vi "store-can-data.vi"(4 "CAN frame":T2 {"payload" format="%x"; "timestamp" format="%<%.7X\n%x>T"; "type" items=["CAN Data"=0, "CAN Remote"=1, "CAN Bus Error"=2, "J1939 Data"=192, "Delay"=224, "Log Trigger"=225, "Start Trigger"=226]; "identifier" format="%x"}, 6 "id":u32 format="%.0x", 7 "child.tags":string[](array[string]), 8 "error in (no error)":errorcluster, 9 "tag":string, 10 "frame.type":T1, 11 "CANtable in":refnum<class "bAPPdata.lvclass">) -> (0 "error out":errorcluster, 3 "CANtable out":refnum<class "bAPPdata.lvclass">)   [LabVIEW 2015, in "bAPPdata.lvclass"]
uses:
  bAPPdata.lvclass
  <vilib>/xnet/xnet.llb/XNET Frame CAN.ctl
  <vilib>/xnet/xnet.llb/XNET Frame Type CAN.ctl
  subs/frame.type.ctl
  bAPPdata.lvclass/bAPPdata.ctl
  table-contents.ctl
  nMsgData.ctl
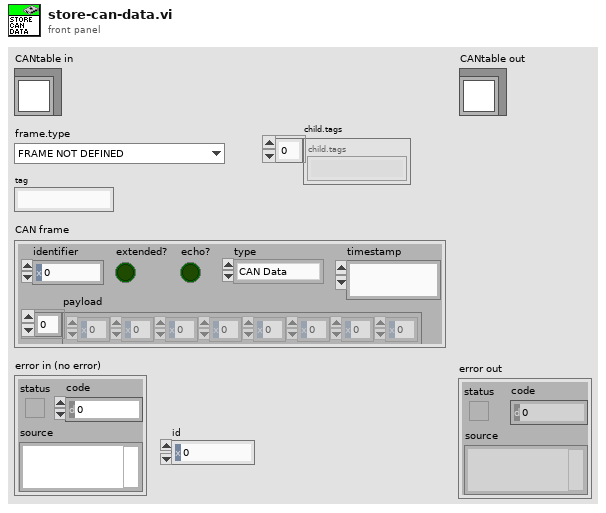
[diagram p1: front panel]
types:
  T1 = typedef "frame.type.ctl" = enum16{"FRAME NOT DEFINED", "DUT OUTPUT FRAME", "DUT INPUT FRAME"}
  T2 = typedef "XNET Frame CAN.ctl" = cluster{"timestamp":timestamp, "payload":u8[], "identifier":u32, "type":T3, "extended?":bool, "echo?":bool}
  T3 = typedef "XNET Frame Type CAN.ctl" = u8
  T4 = typedef "bAPPdata.lvclass/table-contents.ctl" = cluster{"id":u32, "tag":string, "frame.type":T1, "last.frame":T2, "tMsgData":T5, "child.tags":string[], "bit-payload":bool[]}
  T5 = typedef "nMsgData.ctl" = cluster{"dwID":u32, "count":u32, "dwCycleTime":dbl, "dwTime":dbl, "new msg":bool}
  T6 = typedef "bAPPdata.lvclass/table-data.ctl" = T4[]
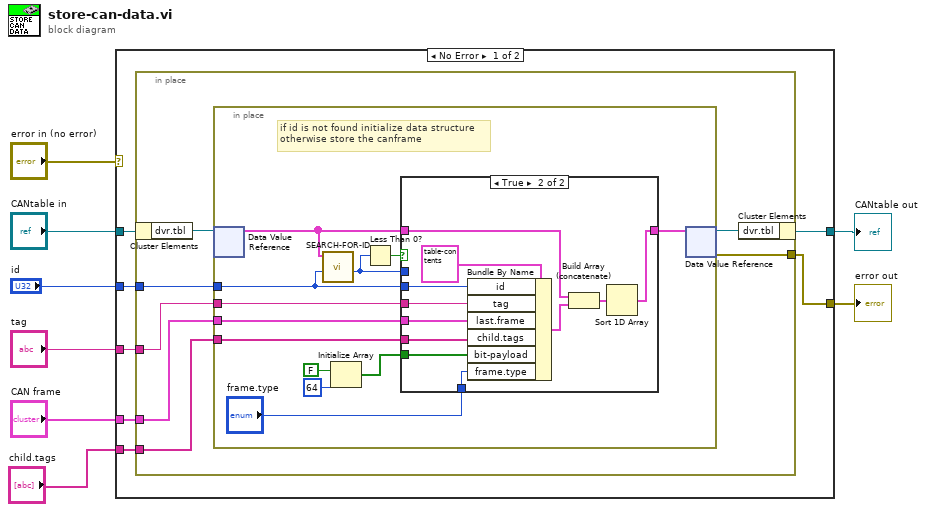
[diagram p0: block diagram]
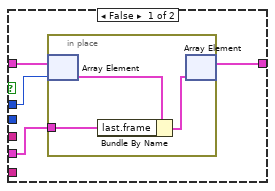
[diagram p2: hidden frame]
diagram:
  n1 = case shown="No Error" "error in (no error)" {
    selector: "error in (no error)" -> [_ w54]
    tunnel: [w12 w54] -> w7
    tunnel: [w14 w53] -> w5
    tunnel: "CANtable in" -> [w15 w53]
    tunnel: "id" -> [w13 _]
    tunnel: "CAN frame" -> [w11 _]
    tunnel: "tag" -> [w10 _]
    tunnel: "child.tags" -> [w9 _]
    frame No Error {
      n2 = in-place {
        in-place-border: [w20] -> w12
        in-place-border: w13 -> [w19]
        in-place-border: w11 -> [w18]
        in-place-border: w10 -> [w17]
        in-place-border: w9 -> [w16]
        n3 = in-place-cluster #1(w15) -> ("dvr.tbl"=w22:refnum<data-value>)
        n4 = in-place {
          in-place-border: w19 -> [w34]
          in-place-border: w18 -> [w33]
          in-place-border: w17 -> [w32]
          in-place-border: w16 -> [w24]
          # "if id is not found initialize data structure\notherwise store the canframe"
          n5 = in-place-dvr #2(w22) -> (w29:T6)  [unwired: 1 out]
          n6 = call "SEARCH-FOR-ID.vi"("ID"=w34, "tbl.list"=w29) -> ("idx"=w30:i32)  [unwired: 8 in, 1 out]
          n7 = Initialize Array(FALSE, 64 ("dimension size")) -> (w25:bool[])
          n8 = Less Than 0?(x=w30) -> (x < 0?=w31:bool)
          n9 = case shown="True" w31 {
            tunnel: w34 -> [_ w47]
            tunnel: [w37 w50] -> w28
            tunnel: w29 -> [w38 w52]
            tunnel: w33 -> [w36 w46]
            tunnel: w32 -> [_ w45]
            tunnel: w30 -> [w35 _]
            tunnel: w24 -> [_ w44]
            tunnel: w25 -> [_ w43]
            tunnel: "frame.type" -> [_ w42]
            frame False {
              n10 = in-place {
                in-place-border: w36 -> [w39]
                n11 = in-place-array #3(w38, w35) -> (w41:T4)
                n12 = Bundle By Name(cluster=w41, "last.frame"=w39) -> (w40:T4)
                n13 = in-place-array #3(w40) -> (w37:T6)  [unwired: 1 out]
              }
            }
            frame True {
              n14 = Bundle By Name(cluster=T4 {"id"=0, "tag"="", "frame.type"=enum."FRAME NOT DEFINED", "last.frame"={"timestamp"=timestamp(0 s since 1904-01-01), "payload"=[], "identifier"=0, "type"=0, "extended?"=FALSE, "echo?"=FALSE}, "tMsgData"={"dwID"=0, "count"=0, "dwCycleTime"=0.0, "dwTime"=0.0, "new msg"=FALSE}, "child.tags"=[], "bit-payload"=[]} ("tbl.cnts"), "id"=w47, "tag"=w45, "last.frame"=w46, "child.tags"=w44, "bit-payload"=w43, "frame.type"=w42) -> (w48:T4)
              n15 = Build Array (concatenate)(w52, w48) -> (w51:T6)
              n16 = Sort 1D Array(array=w51) -> (sorted array=w50:T6)
            }
          }
          n17 = in-place-dvr #2(w28) -> (w21:refnum<data-value>, w20:errorcluster)
        }
        n18 = in-place-cluster #1("dvr.tbl"=w21) -> (w14:refnum<class "bAPPdata.lvclass">)
      }
    }
    frame Error {
    }
  }
  "error out" <- w7
  "CANtable out" <- w5
